vi "addSimulatorDewesoft.vi"(8 "error in (no error)":errorcluster, 10 "IDevice in":refnum<class "IDevice.lvclass">, 11 "IInstance in":refnum<class "IInstance.lvclass">) -> (0 "error out":errorcluster, 2 "IDevice out":refnum<class "IDevice.lvclass">, 3 "IInstance out":refnum<class "IInstance.lvclass">)   [LabVIEW 2022 SP3, in "openDAQ.lvlib" / "daqUtils.lvlib"]
uses:
  daqUtils.lvlib
  IInstance/IInstance.lvclass
  IDevice/IDevice.lvclass
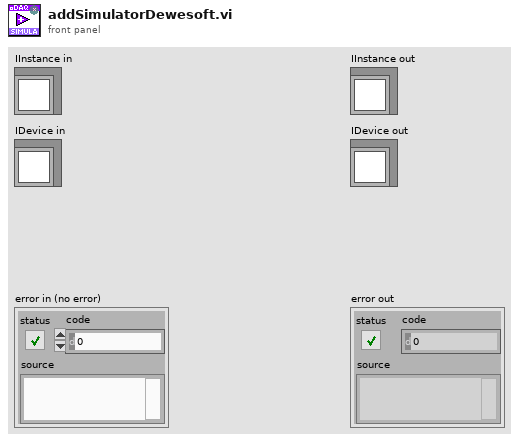
[diagram p1: front panel]
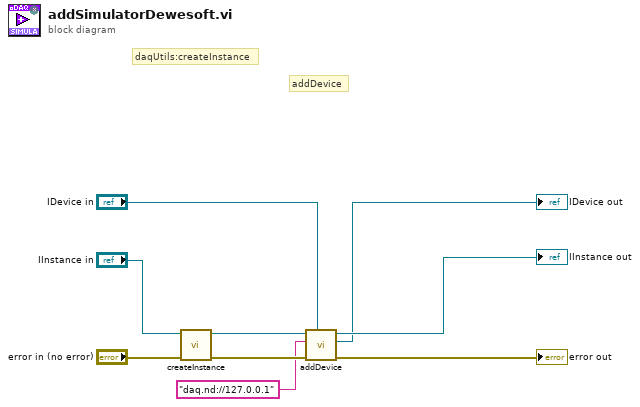
[diagram p0: block diagram]
diagram:
  # "addDevice"
  # "daqUtils:createInstance"
  n1 = call "createInstance.vi"("error in (no error)"="error in (no error)", "IInstance in"="IInstance in") -> ("error out"=w9:errorcluster, "IInstance out"=w1:refnum<class "IInstance.lvclass">)  [unwired: 8 in]
  n2 = call "addDevice.vi"("ConnectedDevice In"="IDevice in", "error in (no error)"=w9, "ConnectionString in"="daq.nd://127.0.0.1", "IDevice in"=w1) -> ("error out"=→"error out":errorcluster, "ConnectedDevice out"=→"IDevice out":refnum<class "IDevice.lvclass">, "IDevice out"=→"IInstance out":refnum<class "IInstance.lvclass">)  [unwired: 5 in]
